vi "UHR-Fleezers Control (host) - Lorentz v3.vi"() -> ()   [LabVIEW 2014] (continued)
                                }
                                frame #3 {
                                n2585 = for {
                                N: 4 -> [_]
                                n2586 = flat-sequence {
                                frame #0 {
                                n2587 = Wait (ms)(milliseconds to wait=u32 500) -> ()  [unwired: 1 out]
                                }
                                frame #1 {
                                n2588 = local read "Action (%)"() -> (w3916:dbl)
                                n2589 = Absolute Value(x=w3916) -> (abs(x)=w3915:dbl)
                                n2590 = Greater?(x=w3915, y=70.0) -> (0:w3913:bool)
                                n2591 = property on="Remove Action Offset" class="Bool (strict)"("Val(Sgnl)"=w3913) -> ()  [unwired: 2 in, 2 out]
                                }
                                }
                                }
                                }
                                frame #4 {
                                n2592 = Wait (ms)(milliseconds to wait=u32 500) -> ()  [unwired: 1 out]
                                }
                                frame #5 {
                                n2593 = local read "Shift confocal"() -> (w3921:bool)
                                n2594 = local read "Mean"() -> (w3924:dbl)
                                n2595 = Greater?(x=w3924, y=11.0) -> (0:w3920:bool)
                                n2596 = Not(x=w3920) -> (.not. x?=w3919:bool)
                                n2597 = And(x=w3920, y=w3921) -> (x .and. y?=w3922:bool)
                                n2598 = And(x=w3919, y=w3921) -> (x .and. y?=w3918:bool)
                                n2599 = case shown="True" w3922 {
                                frame False {
                                }
                                frame True {
                                n2600 = local read "Confocal X 2 (V)"() -> (w3927:dbl)
                                n2601 = local read "Confocal Y 2 (V)"() -> (w3928:dbl)
                                n2602 = property on="AO2" class="Slide (strict)"("Val(Sgnl)"=w3927) -> ()  [unwired: 2 in, 2 out]
                                n2603 = property on="AO1" class="Slide (strict)"("Val(Sgnl)"=w3928) -> ()  [unwired: 2 in, 2 out]
                                }
                                }
                                n2604 = case shown="True" w3918 {
                                frame False {
                                }
                                frame True {
                                n2605 = local read "Confocal Y 1 (V)"() -> (w3926:dbl)
                                n2606 = local read "Confocal X 1 (V)"() -> (w3925:dbl)
                                n2607 = property on="AO1" class="Slide (strict)"("Val(Sgnl)"=w3926) -> ()  [unwired: 2 in, 2 out]
                                n2608 = property on="AO2" class="Slide (strict)"("Val(Sgnl)"=w3925) -> ()  [unwired: 2 in, 2 out]
                                }
                                }
                                }
                                frame #6 {
                                n2609 = Wait (ms)(milliseconds to wait=u32 1500) -> ()  [unwired: 1 out]
                                }
                                frame #7 {
                                n2610 = property on="Rem fb disp offset" class="Bool (strict)"("Val(Sgnl)"=TRUE ("Value (Signaling)")) -> ()  [unwired: 2 in, 2 out]
                                }
                                }
                                }
                                frame True {
                                n2611 = flat-sequence {
                                tunnel: w3931 -> [w3932]
                                frame #0 {
                                n2612 = property on="Trap Delta (MHz)" class="DigNum (strict)"("Val(Sgnl)"=w3932) -> ()  [unwired: 2 in, 2 out]
                                }
                                frame #1 {
                                n2613 = Wait (ms)(milliseconds to wait=u32 500) -> ()  [unwired: 1 out]
                                }
                                frame #2 {
                                n2614 = local read "Shift confocal"() -> (w3938:bool)
                                n2615 = local read "Mean"() -> (w3939:dbl)
                                n2616 = Greater?(x=w3939, y=11.0) -> (0:w3937:bool)
                                n2617 = And(x=w3937, y=w3938) -> (x .and. y?=w3935:bool)
                                n2618 = Not(x=w3937) -> (.not. x?=w3936:bool)
                                n2619 = And(x=w3936, y=w3938) -> (x .and. y?=w3934:bool)
                                n2620 = case shown="True" w3935 {
                                frame False {
                                }
                                frame True {
                                n2621 = local read "Confocal Y 2 (V)"() -> (w3944:dbl)
                                n2622 = local read "Confocal X 2 (V)"() -> (w3943:dbl)
                                n2623 = property on="AO1" class="Slide (strict)"("Val(Sgnl)"=w3944) -> ()  [unwired: 2 in, 2 out]
                                n2624 = property on="AO2" class="Slide (strict)"("Val(Sgnl)"=w3943) -> ()  [unwired: 2 in, 2 out]
                                }
                                }
                                n2625 = case shown="True" w3934 {
                                frame False {
                                }
                                frame True {
                                n2626 = local read "Confocal Y 1 (V)"() -> (w3942:dbl)
                                n2627 = local read "Confocal X 1 (V)"() -> (w3941:dbl)
                                n2628 = property on="AO2" class="Slide (strict)"("Val(Sgnl)"=w3941) -> ()  [unwired: 2 in, 2 out]
                                n2629 = property on="AO1" class="Slide (strict)"("Val(Sgnl)"=w3942) -> ()  [unwired: 2 in, 2 out]
                                }
                                }
                                }
                                }
                                }
                                }
                                }
                                }
                                }
                                }
                                n2630 = local read "Time (s)"() -> (w3879:dbl)
                                n2631 = Subtract(x=w3880, y=w3879) -> (x-y=w3891:dbl)
                                n2632 = Number To Decimal String(number=w3891, width (-)=i16 0) -> (decimal integer string=w3889:string)
                                n2633 = Concatenate Strings(w3889, " s fluorescence event") -> (w3886:string)
                                n2634 = local read "Messages"() -> (w3887:string)
                                n2635 = local write "Duration (s)"(w3891) -> ()
                                n2636 = call "Update messages.vi"("Message to add"=w3886, "Old message string"=w3887) -> ("New message string"=w3885:string)
                                n2637 = local write "Messages"(w3885) -> ()
                                n2638 = call <vilib>:"Beep.vi"() -> ()  [unwired: 12 in]
                                n2639 = local write "Reset Force"(FALSE ("Force Reset")) -> ()
                                n2640 = local write "Fl. High"(TRUE ("Fl. High")) -> ()
                                n2641 = local write "Waiting"(TRUE ("Waiting")) -> ()
                                }
                                }
                                n2642 = node-c288() -> ()  [unwired: 1 in, 1 out]
                                }
                                n2643 = node-c288(w3858) -> ()  [unwired: 1 out]
                                }
                              }
                            }
                          }
                          n2644 = local read "Trap Delta (MHz)"() -> (w3770:dbl)
                          n2645 = local read "Trap Pos FB SP"() -> (w3768:fxp<+/-,16,1>)
                        }
                      }
                    }
                    frame True {
                      n2646 = flat-sequence {
                        tunnel: w3955 -> [w3965]
                        tunnel: [w3965] -> w3959
                        tunnel: w3958 -> [w3964]
                        tunnel: [w3964] -> w3957
                        tunnel: [w3963] -> w3956
                        tunnel: w3954 -> [w3962]
                        tunnel: [w3961] -> w3953
                        tunnel: w3950 -> [w3960]
                        tunnel: [w3960] -> w3949
                        tunnel: w3959 -> [w4035]
                        tunnel: w3957 -> [w4034]
                        tunnel: w3956 -> [w4033]
                        tunnel: w3953 -> [w4032]
                        tunnel: w3949 -> [w4031]
                        tunnel: [w4032] -> w3952
                        frame #0 {
                          n2647 = call <vilib>:"Beep.vi"() -> ()  [unwired: 3 in, 9 out]
                          n2648 = local write "Waiting"(FALSE ("Waiting")) -> ()
                          n2649 = Increment(x=w3962) -> (x+1=w3961:u8)
                          n2650 = case shown="\"Image\"" w3964 {
                            tunnel: w3961 -> [_ _ w3971]
                            frame "Image" {
                              n2651 = property on="Confocal Image" class="Bool (strict)"("Val(Sgnl)"=TRUE ("Value (Signaling)")) -> ()  [unwired: 2 in, 2 out]
                            }
                            frame "Alarm", Default {
                            }
                            frame "Yank" {
                              n2652 = flat-sequence {
                                tunnel: w3971 -> [w3974]
                                tunnel: [w3973] -> w3970
                                tunnel: ["N Array El"] -> w3969
                                tunnel: w3970 -> [w3988]
                                tunnel: w3969 -> [w3984]
                                frame #0 {
                                n2653 = Multiply(x="Yank Delay (s)", y=1000.0) -> (x*y=w3977:dbl)
                                n2654 = Quotient & Remainder(x=w3974, y="N Array El") -> (x-y*floor(x/y)=w3973:u8)  [unwired: 1 out]
                                n2655 = Wait (ms)(milliseconds to wait=w3977) -> ()  [unwired: 1 out]
                                }
                                frame #1 {
                                n2656 = Random Number (0-1)() -> (number: 0 to 1=w3985:dbl)
                                n2657 = Multiply(x=w3984, y=w3985) -> (x*y=w3983:dbl)
                                n2658 = Round Toward -Infinity(1:w3983) -> (0:w3982:dbl)
                                n2659 = Select(t=w3982, s="Random Choice", f=w3988) -> (s? t:f=w3986:dbl)
                                n2660 = Select(t="Yank to Trap Delta (MHz)", s="Yank to which?", f="Yank to SP") -> (s? t:f=w3979:dbl[])
                                n2661 = Index Array(array=w3979, index=w3986) -> (element=w3989:dbl)
                                n2662 = case shown="False" "Yank to which?" {
                                tunnel: w3989 -> [w3990 w4016]
                                frame False {
                                n2663 = flat-sequence {
                                tunnel: w3990 -> [w3991]
                                frame #0 {
                                n2664 = property on="Trap Pos FB SP" class="DigNum (strict)"("Val(Sgnl)"=w3991) -> ()  [unwired: 2 in, 2 out]
                                }
                                frame #1 {
                                n2665 = Wait (ms)(milliseconds to wait=u32 700) -> ()  [unwired: 1 out]
                                }
                                frame #2 {
                                n2666 = local read "Action (%)"() -> (w3996:dbl)
                                n2667 = Absolute Value(x=w3996) -> (abs(x)=w3995:dbl)
                                n2668 = Greater?(x=w3995, y=70.0) -> (0:w3993:bool)
                                n2669 = property on="Remove Action Offset" class="Bool (strict)"("Val(Sgnl)"=w3993) -> ()  [unwired: 2 in, 2 out]
                                }
                                frame #3 {
                                n2670 = for {
                                N: 4 -> [_]
                                n2671 = flat-sequence {
                                frame #0 {
                                n2672 = Wait (ms)(milliseconds to wait=u32 500) -> ()  [unwired: 1 out]
                                }
                                frame #1 {
                                n2673 = local read "Action (%)"() -> (w4002:dbl)
                                n2674 = Absolute Value(x=w4002) -> (abs(x)=w4001:dbl)
                                n2675 = Greater?(x=w4001, y=70.0) -> (0:w3999:bool)
                                n2676 = property on="Remove Action Offset" class="Bool (strict)"("Val(Sgnl)"=w3999) -> ()  [unwired: 2 in, 2 out]
                                }
                                }
                                }
                                }
                                frame #4 {
                                n2677 = local read "Shift confocal"() -> (w4006:bool)
                                n2678 = local read "Mean"() -> (w4009:dbl)
                                n2679 = Greater?(x=w4009, y=11.0) -> (0:w4005:bool)
                                n2680 = Not(x=w4005) -> (.not. x?=w4004:bool)
                                n2681 = And(x=w4004, y=w4006) -> (x .and. y?=w4003:bool)
                                n2682 = And(x=w4005, y=w4006) -> (x .and. y?=w4007:bool)
                                n2683 = case shown="True" w4007 {
                                frame False {
                                }
                                frame True {
                                n2684 = local read "Confocal X 2 (V)"() -> (w4012:dbl)
                                n2685 = local read "Confocal Y 2 (V)"() -> (w4013:dbl)
                                n2686 = property on="AO2" class="Slide (strict)"("Val(Sgnl)"=w4012) -> ()  [unwired: 2 in, 2 out]
                                n2687 = property on="AO1" class="Slide (strict)"("Val(Sgnl)"=w4013) -> ()  [unwired: 2 in, 2 out]
                                }
                                }
                                n2688 = case shown="True" w4003 {
                                frame False {
                                }
                                frame True {
                                n2689 = local read "Confocal X 1 (V)"() -> (w4010:dbl)
                                n2690 = local read "Confocal Y 1 (V)"() -> (w4011:dbl)
                                n2691 = property on="AO1" class="Slide (strict)"("Val(Sgnl)"=w4011) -> ()  [unwired: 2 in, 2 out]
                                n2692 = property on="AO2" class="Slide (strict)"("Val(Sgnl)"=w4010) -> ()  [unwired: 2 in, 2 out]
                                }
                                }
                                }
                                frame #5 {
                                n2693 = Wait (ms)(milliseconds to wait=u32 1500) -> ()  [unwired: 1 out]
                                }
                                frame #6 {
                                n2694 = property on="Rem fb disp offset" class="Bool (strict)"("Val(Sgnl)"=TRUE ("Value (Signaling)")) -> ()  [unwired: 2 in, 2 out]
                                }
                                }
                                }
                                frame True {
                                n2695 = flat-sequence {
                                tunnel: w4016 -> [w4017]
                                frame #0 {
                                n2696 = property on="Trap Delta (MHz)" class="DigNum (strict)"("Val(Sgnl)"=w4017) -> ()  [unwired: 2 in, 2 out]
                                }
                                frame #1 {
                                n2697 = Wait (ms)(milliseconds to wait=u32 500) -> ()  [unwired: 1 out]
                                }
                                frame #2 {
                                n2698 = local read "Shift confocal"() -> (w4021:bool)
                                n2699 = local read "Mean"() -> (w4019:dbl)
                                n2700 = Greater?(x=w4019, y=11.0) -> (0:w4022:bool)
                                n2701 = Not(x=w4022) -> (.not. x?=w4023:bool)
                                n2702 = And(x=w4023, y=w4021) -> (x .and. y?=w4025:bool)
                                n2703 = And(x=w4022, y=w4021) -> (x .and. y?=w4024:bool)
                                n2704 = case shown="True" w4024 {
                                frame False {
                                }
                                frame True {
                                n2705 = local read "Confocal Y 2 (V)"() -> (w4029:dbl)
                                n2706 = local read "Confocal X 2 (V)"() -> (w4028:dbl)
                                n2707 = property on="AO1" class="Slide (strict)"("Val(Sgnl)"=w4029) -> ()  [unwired: 2 in, 2 out]
                                n2708 = property on="AO2" class="Slide (strict)"("Val(Sgnl)"=w4028) -> ()  [unwired: 2 in, 2 out]
                                }
                                }
                                n2709 = case shown="True" w4025 {
                                frame False {
                                }
                                frame True {
                                n2710 = local read "Confocal X 1 (V)"() -> (w4026:dbl)
                                n2711 = local read "Confocal Y 1 (V)"() -> (w4027:dbl)
                                n2712 = property on="AO2" class="Slide (strict)"("Val(Sgnl)"=w4026) -> ()  [unwired: 2 in, 2 out]
                                n2713 = property on="AO1" class="Slide (strict)"("Val(Sgnl)"=w4027) -> ()  [unwired: 2 in, 2 out]
                                }
                                }
                                }
                                }
                                }
                                }
                                }
                              }
                            }
                          }
                          n2714 = local read "Time (s)"() -> (w3963:dbl)
                          "Fl. High" <- TRUE ("Yanking")
                        }
                        frame #1 {
                          n2715 = local read "Auto F Reset"() -> (w4030:bool)
                          n2716 = case shown="True" w4030 {
                            tunnel: w4035 -> [_ w4039]
                            tunnel: w4034 -> [_ w4038]
                            tunnel: w4033 -> [_ w4037]
                            tunnel: w4031 -> [_ w4036]
                            frame False {
                            }
                            frame True {
                              n2717 = node-c288() -> (w4041:T37)  [unwired: 4 out]
                              n2718 = timed-loop {
                                timing: w4041 -> [_]
                                timing-out: [_] -> w4040
                                tunnel: w4039 -> [w4059]
                                tunnel: w4038 -> [w4058]
                                tunnel: w4037 -> [w4057]
                                tunnel: w4036 -> [w4056]
                                stop <- w4042 stop-if-true
                                n2719 = node-c288() -> ()  [unwired: 2 out]
                                n2720 = local read "Fl. Delta Thresh. (kHz)"() -> (w4050:dbl)
                                n2721 = local read "Fl. Triggered..."() -> (w4055:bool)
                                n2722 = local read "Delta Fl. 1"() -> (w4046:dbl)
                                n2723 = local read "Delta Fl. 2"() -> (w4044:dbl)
                                n2724 = local read "Stop All"() -> (w4053:bool)
                                n2725 = local read "APD to Watch"() -> (w4045:bool)
                                n2726 = Select(t=w4046, s=w4045, f=w4044) -> (s? t:f=w4043:dbl)
                                n2727 = Not(x=w4055) -> (.not. x?=w4054:bool)
                                n2728 = Multiply(x=w4050, y=1000.0) -> (x*y=w4049:dbl)
                                n2729 = Negate(x=w4049) -> (-x=w4048:dbl)
                                n2730 = Less?(x=w4043, y=w4048) -> (x < y?=w4052:bool)
                                n2731 = Compound Arithmetic op=OR(w4052, w4053, w4054, "Reset Force") -> (w4042:bool)
                                n2732 = case shown="True" w4042 {
                                tunnel: w4059 -> [_ w4074]
                                tunnel: w4058 -> [_ w4073]
                                tunnel: w4057 -> [_ w4063]
                                tunnel: w4056 -> [_ w4065]
                                frame False {
                                }
                                frame True {
                                n2733 = local read "Time (s)"() -> (w4064:dbl)
                                n2734 = case shown="\"Yank\"" w4073 {
                                tunnel: w4074 -> [_ w4077]
                                tunnel: w4065 -> [_ w4075]
                                frame "Image", Default {
                                }
                                frame "Yank" {
                                n2735 = flat-sequence {
                                tunnel: [w4083] -> w4078
                                tunnel: w4077 -> [w4083]
                                tunnel: [w4079] -> w4076
                                tunnel: w4075 -> [w4079]
                                tunnel: w4078 -> [w4086]
                                tunnel: w4076 -> [w4084]
                                frame #0 {
                                n2736 = local read "Yank Delay (s)"() -> (w4082:dbl)
                                n2737 = Multiply(x=w4082, y=1000.0) -> (x*y=w4080:dbl)
                                n2738 = Wait (ms)(milliseconds to wait=w4080) -> ()  [unwired: 1 out]
                                }
                                frame #1 {
                                n2739 = local read "Yank to which?"() -> (w4085:bool)
                                n2740 = case shown="False" w4085 {
                                tunnel: w4086 -> [_ w4113]
                                tunnel: w4084 -> [w4087 _]
                                frame False {
                                n2741 = flat-sequence {
                                tunnel: w4087 -> [w4088]
                                frame #0 {
                                n2742 = property on="Trap Pos FB SP" class="DigNum (strict)"("Val(Sgnl)"=w4088) -> ()  [unwired: 2 in, 2 out]
                                }
                                frame #1 {
                                n2743 = Wait (ms)(milliseconds to wait=u32 700) -> ()  [unwired: 1 out]
                                }
                                frame #2 {
                                n2744 = local read "Action (%)"() -> (w4093:dbl)
                                n2745 = Absolute Value(x=w4093) -> (abs(x)=w4092:dbl)
                                n2746 = Greater?(x=w4092, y=70.0) -> (0:w4090:bool)
                                n2747 = property on="Remove Action Offset" class="Bool (strict)"("Val(Sgnl)"=w4090) -> ()  [unwired: 2 in, 2 out]
                                }
                                frame #3 {
                                n2748 = for {
                                N: 4 -> [_]
                                n2749 = flat-sequence {
                                frame #0 {
                                n2750 = Wait (ms)(milliseconds to wait=u32 500) -> ()  [unwired: 1 out]
                                }
                                frame #1 {
                                n2751 = local read "Action (%)"() -> (w4099:dbl)
                                n2752 = Absolute Value(x=w4099) -> (abs(x)=w4098:dbl)
                                n2753 = Greater?(x=w4098, y=70.0) -> (0:w4096:bool)
                                n2754 = property on="Remove Action Offset" class="Bool (strict)"("Val(Sgnl)"=w4096) -> ()  [unwired: 2 in, 2 out]
                                }
                                }
                                }
                                }
                                frame #4 {
                                n2755 = local read "Shift confocal"() -> (w4104:bool)
                                n2756 = local read "Mean"() -> (w4106:dbl)
                                n2757 = Greater?(x=w4106, y=11.0) -> (0:w4103:bool)
                                n2758 = Not(x=w4103) -> (.not. x?=w4102:bool)
                                n2759 = And(x=w4103, y=w4104) -> (x .and. y?=w4101:bool)
                                n2760 = And(x=w4102, y=w4104) -> (x .and. y?=w4100:bool)
                                n2761 = case shown="True" w4101 {
                                frame False {
                                }
                                frame True {
                                n2762 = local read "Confocal Y 2 (V)"() -> (w4110:dbl)
                                n2763 = local read "Confocal X 2 (V)"() -> (w4109:dbl)
                                n2764 = property on="AO2" class="Slide (strict)"("Val(Sgnl)"=w4109) -> ()  [unwired: 2 in, 2 out]
                                n2765 = property on="AO1" class="Slide (strict)"("Val(Sgnl)"=w4110) -> ()  [unwired: 2 in, 2 out]
                                }
                                }
                                n2766 = case shown="True" w4100 {
                                frame False {
                                }
                                frame True {
                                n2767 = local read "Confocal X 1 (V)"() -> (w4107:dbl)
                                n2768 = local read "Confocal Y 1 (V)"() -> (w4108:dbl)
                                n2769 = property on="AO1" class="Slide (strict)"("Val(Sgnl)"=w4108) -> ()  [unwired: 2 in, 2 out]
                                n2770 = property on="AO2" class="Slide (strict)"("Val(Sgnl)"=w4107) -> ()  [unwired: 2 in, 2 out]
                                }
                                }
                                }
                                frame #5 {
                                n2771 = Wait (ms)(milliseconds to wait=u32 1500) -> ()  [unwired: 1 out]
                                }
                                frame #6 {
                                n2772 = property on="Rem fb disp offset" class="Bool (strict)"("Val(Sgnl)"=TRUE ("Value (Signaling)")) -> ()  [unwired: 2 in, 2 out]
                                }
                                }
                                }
                                frame True {
                                n2773 = flat-sequence {
                                tunnel: w4113 -> [w4114]
                                frame #0 {
                                n2774 = property on="Trap Delta (MHz)" class="DigNum (strict)"("Val(Sgnl)"=w4114) -> ()  [unwired: 2 in, 2 out]
                                }
                                frame #1 {
                                n2775 = Wait (ms)(milliseconds to wait=u32 500) -> ()  [unwired: 1 out]
                                }
                                frame #2 {
                                n2776 = local read "Shift confocal"() -> (w4120:bool)
                                n2777 = local read "Mean"() -> (w4122:dbl)
                                n2778 = Greater?(x=w4122, y=11.0) -> (0:w4119:bool)
                                n2779 = Not(x=w4119) -> (.not. x?=w4118:bool)
                                n2780 = And(x=w4119, y=w4120) -> (x .and. y?=w4117:bool)
                                n2781 = And(x=w4118, y=w4120) -> (x .and. y?=w4116:bool)
                                n2782 = case shown="True" w4117 {
                                frame False {
                                }
                                frame True {
                                n2783 = local read "Confocal Y 2 (V)"() -> (w4126:dbl)
                                n2784 = local read "Confocal X 2 (V)"() -> (w4125:dbl)
                                n2785 = property on="AO2" class="Slide (strict)"("Val(Sgnl)"=w4125) -> ()  [unwired: 2 in, 2 out]
                                n2786 = property on="AO1" class="Slide (strict)"("Val(Sgnl)"=w4126) -> ()  [unwired: 2 in, 2 out]
                                }
                                }
                                n2787 = case shown="True" w4116 {
                                frame False {
                                }
                                frame True {
                                n2788 = local read "Confocal Y 1 (V)"() -> (w4124:dbl)
                                n2789 = local read "Confocal X 1 (V)"() -> (w4123:dbl)
                                n2790 = property on="AO2" class="Slide (strict)"("Val(Sgnl)"=w4123) -> ()  [unwired: 2 in, 2 out]
                                n2791 = property on="AO1" class="Slide (strict)"("Val(Sgnl)"=w4124) -> ()  [unwired: 2 in, 2 out]
                                }
                                }
                                }
                                }
                                }
                                }
                                }
                                }
                                }
                                }
                                n2792 = local read "Messages"() -> (w4072:string)
                                n2793 = Subtract(x=w4064, y=w4063) -> (x-y=w4070:dbl)
                                "Duration (s)" <- w4070
                                n2794 = Number To Decimal String(number=w4070, width (-)=i16 0) -> (decimal integer string=w4068:string)
                                n2795 = Concatenate Strings(w4068, " s fluorescence event." ("string")) -> (w4066:string)
                                n2796 = call "Update messages.vi"("Message to add"=w4066, "Old message string"=w4072) -> ("New message string"=w4071:string)
                                n2797 = local write "Reset Force"(FALSE ("Reset Force")) -> ()
                                n2798 = local write "Waiting"(TRUE ("Waiting")) -> ()
                                n2799 = local write "Messages"(w4071) -> ()
                                n2800 = local write "Fl. High"(FALSE ("Fl. High")) -> ()
                                n2801 = call <vilib>:"Beep.vi"() -> ()  [unwired: 3 in, 9 out]
                                }
                                }
                                n2802 = node-c288() -> ()  [unwired: 2 out]
                              }
                              n2803 = node-c288(w4040) -> ()  [unwired: 1 out]
                            }
                          }
                        }
                      }
                      n2804 = local read "Trap Delta (MHz)"() -> (w3955:dbl)
                      n2805 = local read "Trap Pos FB SP"() -> (w3950:fxp<+/-,16,1>)
                    }
                  }
                }
                frame #1 {
                  n2806 = local read "Stop All"() -> (w4136:bool)
                  n2807 = local read "Fl. Triggered..."() -> (w4134:bool)
                  n2808 = Not(x=w4134) -> (.not. x?=w4135:bool)
                  n2809 = Or(x=w4135, y=w4136) -> (x .or. y?=w4133:bool)
                }
              }
              n2810 = case shown="True" w3727 {
                frame False {
                }
                frame True {
                  n2811 = local read "Confocal Y 1 (V)"() -> (w3737:dbl)
                  n2812 = local read "Confocal X 1 (V)"() -> (w3736:dbl)
                  n2813 = property on="AO2" class="Slide (strict)"("Val(Sgnl)"=w3736) -> ()  [unwired: 2 in, 2 out]
                  n2814 = property on="AO1" class="Slide (strict)"("Val(Sgnl)"=w3737) -> ()  [unwired: 2 in, 2 out]
                }
              }
              n2815 = case shown="True" w3727 {
                frame False {
                }
                frame True {
                  w3735 = FALSE ("Fl. High")
                  n2816 = local write "Waiting"(w3735) -> ()
                  n2817 = local write "Fl. High"(w3735) -> ()
                }
              }
              n2818 = node-c288() -> ()  [unwired: 2 out]
            }
            n2819 = node-c288(w3725) -> ()  [unwired: 1 out]
          }
        }
      }
      event "Start assembly line": Value Change {
        n2820 = event-data() -> ()  [unwired: 7 out]
        n2821 = case shown="True" "Start assembly line" {
          tunnel: w4142 -> [_ w4143]
          frame False {
          }
          frame True {
            n2822 = flat-sequence {
              tunnel: w4143 -> [w4148]
              tunnel: [w4147] -> w4145
              tunnel: w4145 -> [w4180]
              tunnel: [w4179] -> w4144
              tunnel: w4144 -> [w4182]
              tunnel: w4143 -> [w4201]
              frame #0 {
                w4146 = TRUE ("Value (Signaling)")
                n2823 = property on="Green Laser ON" class="Bool (strict)"("Val(Sgnl)"=w4146) -> ()  [unwired: 2 in, 2 out]
                "AL Running" <- w4146
              }
              frame #1 {
                n2824 = node-c288() -> (w4150:T37)  [unwired: 4 in]
                n2825 = timed-loop {
                  timing: w4150 -> [_]
                  timing-out: [_] -> w4149
                  tunnel: w4148 -> [w4158]
                  tunnel: [w4153] -> w4147
                  stop <- w4154 stop-if-true
                  n2826 = node-c288() -> ()  [unwired: 1 in, 1 out]
                  n2827 = local read "APD rates cluster"() -> (w4152:T1)
                  n2828 = Multiply(x="Cy3 Fl.  Thresh. (kHz)", y=1000.0) -> (x*y=w4161:dbl)
                  n2829 = Unbundle By Name(w4152) -> ("APD 1 Rate (Hz)"=w4151:dbl)
                  n2830 = Greater?(x=w4151, y=w4161) -> (0:w4157:bool)
                  n2831 = case shown="True" w4157 {
                    tunnel: w4158 -> [_ w4164]
                    tunnel: [TRUE ("Stage Moving") w4163] -> w4156
                    frame False {
                    }
                    frame True {
                      n2832 = flat-sequence {
                        tunnel: w4164 -> [w4169]
                        tunnel: [w4174] -> w4163
                        frame #0 {
                          n2833 = Multiply(x="AL Delay (s)", y=u32 1000) -> (x*y=w4166:u32)
                          n2834 = Wait (ms)(milliseconds to wait=w4166) -> ()  [unwired: 1 out]
                        }
                        frame #1 {
                          n2835 = property on="Green Laser ON" class="Bool (strict)"("Val(Sgnl)"=FALSE ("Value (Signaling)")) -> ()  [unwired: 2 in, 2 out]
                        }
                        frame #2 {
                          # "upper spot"
                          n2836 = local read "Saved Stage Positions"() -> (w4172:dbl[][])
                          n2837 = local write "Stage Moving"(TRUE ("Stage Moving")) -> ()
                          n2838 = call "move to saved stage position.vi"("Stage VISA resource name in"=w4169, "Position"=5, "Saved Stage Positions"=w4172) -> ("error out"=w4170:errorcluster)  [unwired: 1 in, 1 out]
                          n2839 = local write "Stage Control Serial Error"(w4170) -> ()
                        }
                        frame #3 {
                          w4174 = FALSE ("Stage Moving")
                          n2840 = call <vilib>:"Beep.vi"() -> ()  [unwired: 3 in, 9 out]
                          n2841 = local write "Stage Moving"(w4174) -> ()
                        }
                      }
                    }
                  }
                  n2842 = local read "Stop assembly line"() -> (w4153:bool)
                  n2843 = Not(x=w4156) -> (.not. x?=w4155:bool)
                  n2844 = node-c288() -> ()  [unwired: 1 in, 1 out]
                  n2845 = Or(x=w4155, y=w4153) -> (x .or. y?=w4154:bool)
                }
                n2846 = node-c288(w4149) -> ()  [unwired: 1 out]
              }
              frame #2 {
                n2847 = Not(x=w4180) -> (.not. x?=w4179:bool)
                n2848 = case shown="True" w4179 {
                  frame False {
                  }
                  frame True {
                    n2849 = property on="Red Laser ON" class="Bool (strict)"("Val(Sgnl)"=TRUE ("Value (Signaling)")) -> ()  [unwired: 2 in, 2 out]
                  }
                }
              }
              frame #3 {
                n2850 = node-c288() -> (w4184:T37)  [unwired: 4 in]
                n2851 = timed-loop {
                  timing: w4184 -> [_]
                  timing-out: [_] -> w4183
                  tunnel: [w4187] -> _
                  tunnel: w4182 -> [w4187]
                  stop <- "Stop assembly line" stop-if-true
                  n2852 = node-c288() -> ()  [unwired: 1 in, 1 out]
                  n2853 = local read "APD rates cluster"() -> (w4186:T1)
                  n2854 = Multiply(x="Cy5 Fl.  Thresh. (kHz)", y=1000.0) -> (x*y=w4193:dbl)
                  n2855 = Unbundle By Name(w4186) -> ("APD 2 Rate (Hz)"=w4185:dbl)
                  n2856 = Greater?(x=w4185, y=w4193) -> (0:w4190:bool)
                  n2857 = And(x=w4190, y=w4187) -> (x .and. y?=w4188:bool)
                  n2858 = case shown="True" w4188 {
                    frame False {
                    }
                    frame True {
                      n2859 = property on="Green Laser ON" class="Bool (strict)"("Val(Sgnl)"=TRUE ("Value (Signaling)")) -> ()  [unwired: 2 in, 2 out]
                    }
                  }
                  n2860 = node-c288() -> ()  [unwired: 1 in, 1 out]
                }
                n2861 = node-c288(w4183) -> ()  [unwired: 1 out]
              }
              frame #4 {
                w4200 = FALSE ("Value (Signaling)")
                # "lower spot"
                n2862 = local read "Saved Stage Positions"() -> (w4204:dbl[][])
                n2863 = property on="Red Laser ON" class="Bool (strict)"("Val(Sgnl)"=w4200) -> ()  [unwired: 2 in, 2 out]
                n2864 = property on="Green Laser ON" class="Bool (strict)"("Val(Sgnl)"=w4200) -> ()  [unwired: 2 in, 2 out]
                n2865 = local write "Stage Moving"(TRUE ("Stage Moving")) -> ()
                n2866 = local write "Stop assembly line"(FALSE ("Stop assembly line")) -> ()
                n2867 = call "move to saved stage position.vi"("Stage VISA resource name in"=w4201, "Position"=3, "Saved Stage Positions"=w4204) -> ("error out"=w4203:errorcluster)  [unwired: 1 in, 1 out]
                n2868 = local write "Stage Control Serial Error"(w4203) -> ()
              }
              frame #5 {
                w4206 = FALSE ("Stage Moving")
                n2869 = local write "Stage Moving"(w4206) -> ()
                n2870 = local write "AL Running"(w4206) -> ()
                n2871 = call <vilib>:"Beep.vi"() -> ()  [unwired: 3 in, 9 out]
              }
            }
          }
        }
      }
      event "Stop All": Value Change {
        n2872 = event-data() -> ()  [unwired: 7 out]
        n2873 = local read "Stop All"() -> (w4207:bool)
      }
    }
    n2874 = node-c288() -> ()  [unwired: 2 out]
  }
  n2875 = node-c288(w32) -> ()  [unwired: 1 out]
  n2876 = node-c288(w64) -> ()  [unwired: 1 out]
  n2877 = node-c288(w66) -> ()  [unwired: 1 out]
  n2878 = node-c288(w54) -> ()  [unwired: 1 out]
  n2879 = property on="Saved trap pos" class="WFGraph (strict)"("Visible"=FALSE) -> ()  [unwired: 2 in, 2 out]
  n2880 = property on="Trap Delta Graph" class="WFGraph (strict)"("Visible"=TRUE) -> ()  [unwired: 2 in, 2 out]
  n2881 = disable-structure shown="Disabled" {
    disable-tunnel: w57 -> [w4209 _]
    disable-tunnel: w56 -> [w4208 _]
    frame Disabled {
      n2882 = VISA Close(VISA resource name=w4209, error in (no error)=w4208) -> (error out=w4210:errorcluster)
      n2883 = call <vilib>:"Simple Error Handler.vi"("error in (no error)"=w4210) -> ()  [unwired: 1 in, 8 out]
    }
    frame Enabled {
    }
  }
  n2884 = disable-structure shown="Disabled" {
    disable-tunnel: [w4218 _] -> w18
    disable-tunnel: [w4214 _] -> w17
    disable-tunnel: [w4213 _] -> w16
    disable-tunnel: [w4212 _] -> w15
    disable-tunnel: [w4211 _] -> w14
    frame Disabled {
      # "n samples needed for data"
      n2885 = Unbundle By Name("sound format") -> ("sample rate (S/s)"=w4214:dbl)
      n2886 = call <vilib>:"Sound Output Configure.vi"("number of samples/ch"="number of samples/ch", "sample mode"="sample mode", "sound format"="sound format", "device ID"="device ID") -> ("task ID"=w4218:T51)  [unwired: 6 in, 1 out]
      n2887 = local read "DMA Update Period (s)"() -> (w4215:dbl)
      n2888 = Multiply(x=w4215, y=w4214) -> (x*y=w4213:dbl)
      n2889 = for "Sound time base" {
        N: w4213 -> [_]
        tunnel: [w4222] -> w4216 mode=indexing
        i -> [w4222]
      }
      n2890 = Reciprocal(x=w4214) -> (1/x=w4212:dbl)
      n2891 = Multiply(x=w4216, y=w4212) -> (x*y=w4211:dbl[])
    }
    frame Enabled {
    }
  }
  n2892 = timed-loop "Main data acquisition loop (get data, process data for display, and save data to disk)" {
    tunnel: w13 -> [w4312]
    tunnel: w26 -> [w4311]
    tunnel: [w4571] -> w78
    tunnel: [w4566] -> w77
    timing: w71 -> [_]
    timing-out: [_] -> w70
    tunnel: w48 -> [w4478]
    tunnel: [w4368] -> w19
    tunnel: w18 -> [w4367]
    tunnel: w17 -> [w4365]
    tunnel: w16 -> [w4364]
    tunnel: w15 -> [w4363]
    tunnel: w14 -> [w4362]
    tunnel: w3 -> [w4303]
    tunnel: w2 -> [w4302]
    tunnel: [w4297] -> w1
    stop <- "Stop All" stop-if-true
    w4242 = 2.0
    w4268 = 3276.7
    w4425 = "Initialize"
    # "Cursor control of MCL trap position"
    # "Values for plotting"
    # "Added by Ronen - the limits imposed on amplitudes sent to AOM\nare not explicitly imposed when using intensity feedback. At amplitude of \n~48% FB intensity is ~1.8, if while feedback is on the value passes 1.8, feedback\nis turned off (indication that feedback algorithm overshoots)."
    # "List of channels in order (X or Y only):\nT1 X (mV)\nT2 X (mV)\nT1 X (nm)\nT2 X (nm)\nT1 FX (pN)\nT2 FX (pN)\nPosition Difference (nm)\nAPD1\nAPD2\nAPD3"
    # "T2 sum"
    # "T1 sum"
    n2893 = node-c288() -> ()  [unwired: 2 out]
    n2894 = First Call?() -> (First Call?: T/F=w4438:bool)
    n2895 = Or(x="Reset", y=w4438) -> (x .or. y?=w4439:bool)
    n2896 = Or(x="Start AOD Scan", y="Trap Raster Scan") -> (x .or. y?=w4525:bool)
    n2897 = case "Reset data stream (manual reset or at begining of some rastering and imaging)" shown="True" w4439 {
      tunnel: w4312 -> [w5324 w5332]
      tunnel: w4311 -> [w5323 w5331]
      tunnel: [w5324 w5326] -> w4342
      tunnel: [w5323 w5325] -> w4343
      frame False {
      }
      frame True {
        w5329 = TRUE ("AI to FIFO")
        n2898 = call "reset FPGA DMA.vi"("error in"=w5331, "FPGA VI Reference In"=w5332) -> ("error out"=w5327:errorcluster, "FPGA VI Reference Out"=w5328:T36)
        n2899 = local write "Overflow (data lost)"(FALSE ("Overflow (data lost)")) -> ()
        n2900 = xnode "Read/Write Control"("FPGA VI Reference In"=w5328, "error in"=w5327, "AI to FIFO"=w5329, "APD to FIFO"=w5329) -> ("FPGA VI Reference Out"=w5326:T36, "error out"=w5325:errorcluster)
      }
    }
    n2901 = case "Start active calibration (oscillate traps precisely)" shown="True" "Active Cal" {
      tunnel: w4343 -> [w4674 w4682]
      tunnel: w4342 -> [w4673 w4683]
      tunnel: [w4674 w4679] -> w4341
      tunnel: [w4673 w4680] -> w4340
      frame False {
      }
      frame True {
        w4675 = TRUE ("APD to FIFO")
        n2902 = call "reset FPGA DMA.vi"("error in"=w4682, "FPGA VI Reference In"=w4683) -> ("error out"=w4676:errorcluster, "FPGA VI Reference Out"=w4677:T36)
        n2903 = local write "Active Cal"(FALSE ("Active Cal")) -> ()
        n2904 = local write "Save Calibration"(TRUE ("Save Calibration")) -> ()
        n2905 = xnode "Read/Write Control"("FPGA VI Reference In"=w4677, "error in"=w4676, "AI to FIFO"=w4675, "APD to FIFO"=w4675) -> ("FPGA VI Reference Out"=w4680:T36, "error out"=w4679:errorcluster)
      }
    }
    n2906 = case shown="True" "Read Lateness and Rel Phase" {
      tunnel: w4312 -> [w4898 w4929]
      tunnel: w4311 -> [w4899 w4928]
      tunnel: [w4898 w4900] -> w4264
      tunnel: [w4899 w4901] -> w4514
      frame False {
      }
      frame True {
        n2907 = xnode "Read/Write Control"("FPGA VI Reference In"=w4929, "error in"=w4928) -> ("FPGA VI Reference Out"=w4900:T36, "error out"=w4901:errorcluster, "GI Relative phase"=→"GI relative phase":i16, "Relative phase"=→"Relative phase (AI1)":i16, "AI Late Counter"=→"Late Counter (AI1)":u8, "GI Late Counter"=→"GI Late Counter":u8, "MCL Late Counter"=→"MCL Late Counter":u8, "MCL Relative Phase"=→"Relative Phase (MCL)":i16, "APD Acq Relative Phase"=→"APD Acq Relative Phase":i16, "APD 1 Gate Relative Phase"=→"APD 1 Gate Relative Phase":i16, "APD 2 Gate Relative Phase"=→"APD 2 Gate Relative Phase":i16, "APD Acq Late Counter"=→"APD Acq Late Counter":u8, "APD 1 Gate Late Counter"=→"APD 1 Gate Late Counter":u8, "APD 2 Gate Late Counter"=→"APD 2 Gate Late Counter":u8, "Green FB Relative Phase"=→"Relative phase (Green FB)":i16, "GI Relative phase 2"=→"GI relative phase 2":i16, "GI Late Counter 2"=→"GI Late Counter 2":u8, "Trap Pos FIFO Timeout"=→"Trap Pos FIFO Timeout":u16, "Trap AI FIFO Timeout"=→"Trap AI FIFO Timeout":u16, "RI Late Counter"=→"RI Late Counter":u8, "RI Relative phase"=→"RI relative phase":i16, "Green Late Counter"=→"Green AI Late Counter":u8, "BI Late Counter (AO)"=→"Late Counter (BI AO)":u8, "Blue Late Counter (D)"=→"Late Counter (BI DO)":u8, "BI Relative phase (AO)"=→"Relative phase (BI AO)":i16, "BI Relative phase (D)"=→"Relative phase (BI DO)":i16, "APD 3 Gate Late Counter"=→"APD 3 Gate Late Counter":u8, "APD 3 Gate Relative Phase"=→"APD 3 Gate Relative Phase":i16)
      }
    }
    n2908 = Compound Arithmetic op=OR("Start MCL Scan", "Confocal Image", "Confocal Linescan") -> (w4310:bool)
    n2909 = And(x="Save Data (MCL)", y=w4310) -> (x .and. y?=w4544:bool)
    n2910 = case "Start AOM raster scan" shown="True" w4525 {
      tunnel: w4340 -> [w5183 w5193]
      tunnel: w4341 -> [w5182 w5192]
      tunnel: [w5183 w5186] -> w4547
      tunnel: [w5182 w5185] -> w4546
      frame False {
      }
      frame True {
        n2911 = case shown="True" "Restart DMA? (AOD)" {
          tunnel: [w5222 w5224] -> w5187
          tunnel: [w5221 w5223] -> w5188
          tunnel: w5193 -> [w5222 w5226]
          tunnel: w5192 -> [w5221 w5225]
          frame False {
          }
          frame True {
            n2912 = local write "Overflow (data lost)"(FALSE ("Overflow (data lost)")) -> ()
            n2913 = call "reset FPGA DMA.vi"("error in"=w5225, "FPGA VI Reference In"=w5226) -> ("error out"=w5223:errorcluster, "FPGA VI Reference Out"=w5224:T36)
          }
        }
        n2914 = local write "Trap Raster Scan"(FALSE ("Trap Raster Scan")) -> ()
        n2915 = case shown="True" "Move MCL Also?" {
          tunnel: w5188 -> [w5196 w5216]
          tunnel: w5187 -> [w5197 w5217]
          tunnel: [w5195 w5220] -> w5186
          tunnel: [w5194 w5219] -> w5185
          frame False {
            w5198 = TRUE ("AI to FIFO")
            n2916 = xnode "Read/Write Control"("FPGA VI Reference In"=w5197, "error in"=w5196, "AI to FIFO"=w5198, "APD to FIFO"=w5198, "Start scan"=w5198) -> ("FPGA VI Reference Out"=w5195:T36, "error out"=w5194:errorcluster)
          }
          frame True {
            w5214 = FALSE ("1D or 2D Scan?")
            w5218 = TRUE ("AI to FIFO")
            n2917 = local read "Scan Range (nm)"() -> (w5211:dbl)
            n2918 = local read "Scan steps (AOD)"() -> (w5205:u64)
            n2919 = local read "Total Counts (ticks)"() -> (w5206:u16)
            n2920 = local read "Cycles/step (AOD)"() -> (w5204:u64)
            n2921 = local read "Number of F/B Scans (AOD)"() -> (w5213:u16)
            n2922 = Bundle("Scan Range (nm)"=w5211, "MCL Step Position Ratio"="MCL Step Position Ratio", "MCL/AOM Scale Tweak"="MCL/AOM Scale Tweak", "MCL X Cal (nm/V)"="MCL X Cal (nm/V)", "MCL Step Increment (V_int)"="MCL Step Increment (V_int)", "Total Counts (ticks)"=w5206, "Scan steps (AOD)"=w5205, "Cycles/step (AOD)"=w5204) -> (w5203:T58)  [unwired: 1 in]
            n2923 = call "Calculate MCL scan parameters.vi"("Input parameters"=w5203) -> ("Scan steps(MCL)"=w5202:dbl, "Scan Freq. Increment (MCL)"=w5201:dbl, "MCL Count"=w5200:dbl)
            "MCL Count" <- w5200
            n2924 = xnode "Read/Write Control"("FPGA VI Reference In"=w5217, "error in"=w5216, "Scan steps (MCL)"=w5202, "Number of scans (MCL)"=w5213, "Cycles per step (MCL)"=u64 1, "Scan freq.  increment (MCL)"=w5201, "1D or 2D Scan?"=w5214, "MCL Scan Axis"=w5214, "Cont. Scan (MCL)"=w5214, "MCL count"=w5200) -> ("FPGA VI Reference Out"=w5199:T36, "error out"=w5215:errorcluster)
            n2925 = local write "MCL Scanning"(w5218) -> ()
            n2926 = local write "wait to reset values"(w5218) -> ()
            n2927 = xnode "Read/Write Control"("FPGA VI Reference In"=w5199, "error in"=w5215, "AI to FIFO"=w5218, "APD to FIFO"=w5218, "Start scan"=w5218, "Start scan (MCL)"=w5218) -> ("FPGA VI Reference Out"=w5220:T36, "error out"=w5219:errorcluster)
          }
        }
        "Raster Scanning..." <- TRUE ("Scanning...")
      }
    }
    n2928 = case "Start MCL raster scan" shown="True" w4310 {
      tunnel: w4547 -> [w5111 w5126]
      tunnel: w4546 -> [w5110 w5125]
      tunnel: [w5111 w5121] -> w4477
      tunnel: [w5110 w5120] -> w4476
      tunnel: [FALSE w5119] -> w4530
      tunnel: "Start MCL Scan" -> [_ w5114]
      tunnel: "Confocal Image" -> [_ w5113]
      tunnel: "Confocal Linescan" -> [_ _]
      frame False {
      }
      frame True {
        w5119 = TRUE
        n2929 = case shown="True" "Restart DMA? (MCL)" {
          tunnel: [w5155 w5157] -> w5124
          tunnel: [w5154 w5156] -> w5123
          tunnel: w5126 -> [w5155 w5160]
          tunnel: w5125 -> [w5154 w5159]
          frame False {
          }
          frame True {
            n2930 = call "reset FPGA DMA.vi"("error in"=w5159, "FPGA VI Reference In"=w5160) -> ("error out"=w5156:errorcluster, "FPGA VI Reference Out"=w5157:T36)
            n2931 = local write "Overflow (data lost)"(FALSE ("Overflow (data lost)")) -> ()
          }
        }
        n2932 = case shown="False" w5114 {
          tunnel: w5113 -> [w5129 _]
          frame False {
            n2933 = property on="Confocal Image" class="Bool (strict)"("Value"=FALSE ("Start Confocal Map")) -> ()  [unwired: 2 in, 2 out]
            n2934 = property on="2D or 1D Scan" class="Bool (strict)"("Val(Sgnl)"=w5129) -> ()  [unwired: 2 in, 2 out]
          }
          frame True {
          }
        }
        n2935 = local write "Tab Control 6"(T3."Imaging" ("Tab Control 6")) -> ()
        n2936 = local write "MCL Scanning"(w5119) -> ()
        n2937 = local read "AO2"() -> (w5115:dbl)
        n2938 = local read "AO1"() -> (w5116:dbl)
        n2939 = case shown="True" "Center Scan" {
          tunnel: w5124 -> [w5136 w5153]
          tunnel: w5123 -> [w5135 w5152]
          tunnel: [w5134 w5151] -> w5121
          tunnel: [w5133 w5150] -> w5120
          tunnel: [w5131 w5138] -> w5118
          tunnel: [w5130 w5137] -> w5117
          tunnel: w5116 -> [w5131 w5143]
          tunnel: w5115 -> [w5130 w5142]
          frame False {
            w5132 = TRUE ("AI to FIFO")
            n2940 = xnode "Read/Write Control"("FPGA VI Reference In"=w5136, "error in"=w5135, "AI to FIFO"=w5132, "APD to FIFO"=w5132, "Start scan (MCL)"=w5132) -> ("FPGA VI Reference Out"=w5134:T36, "error out"=w5133:errorcluster)
          }
          frame True {
            w5149 = TRUE ("AI to FIFO")
            n2941 = local read "Actual MCL Inc (V)"() -> (w5146:dbl)
            n2942 = local read "Scan steps (MCL)"() -> (w5145:u64)
            n2943 = local read "Scan lines (y)"() -> (w5144:u64)
            n2944 = local read "2D or 1D Scan"() -> (w5139:bool)
            n2945 = local read "Fast Scan Dir"() -> (w5140:bool)
            n2946 = Bundle("Actual MCL Inc (V)"=w5146, "Scan steps (MCL)"=w5145, "Scan lines (y)"=w5144, "AO1"=w5143, "AO2"=w5142) -> (w5141:T59)  [unwired: 1 in]
            n2947 = call "Center Scan calculation.vi"("2D or 1D Scan"=w5139, "Fast Scan Dir"=w5140, "Input parameters"=w5141) -> ("AO2"=w5137:dbl, "AO1"=w5138:dbl)
            n2948 = call "Volt to I16.vi"("Voltage In"=w5138) -> ("I16 Voltage Out"=w5148:i16)
